vi "13_ВПУравнения.vi"() -> ()   [LabVIEW 2016]
panel:
  out "Y2":dbl
  out "Y1":dbl
  in  "b":dbl
  in  "M":dbl
  in  "X3":dbl
  in  "X2":dbl
  in  "X":dbl
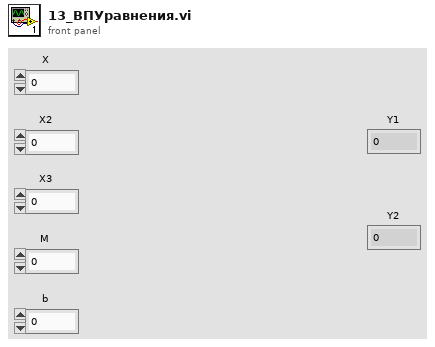
[diagram p1: front panel]
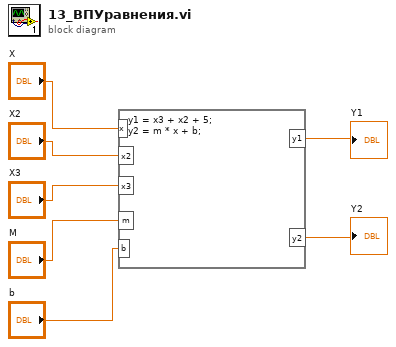
[diagram p0: block diagram]
diagram:
  n1 = formula code="y1 = x3 + x2 + 5;\ny2 = m * x + b;"("x"="X", "x2"="X2", "x3"="X3", "m"="M", "b"="b") -> ("y1"=→"Y1":dbl, "y2"=→"Y2":dbl)
